vi "NorthWest Window Control_Async.vi"(1 "Desired Window Open %":dbl) -> ()   [LabVIEW 2017]
uses:
  Anemometry/Anemometry Sub Vis/Globals/Dynamic_call_global.ph.vi
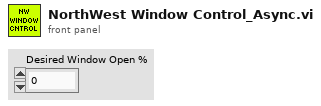
[diagram p1: front panel]
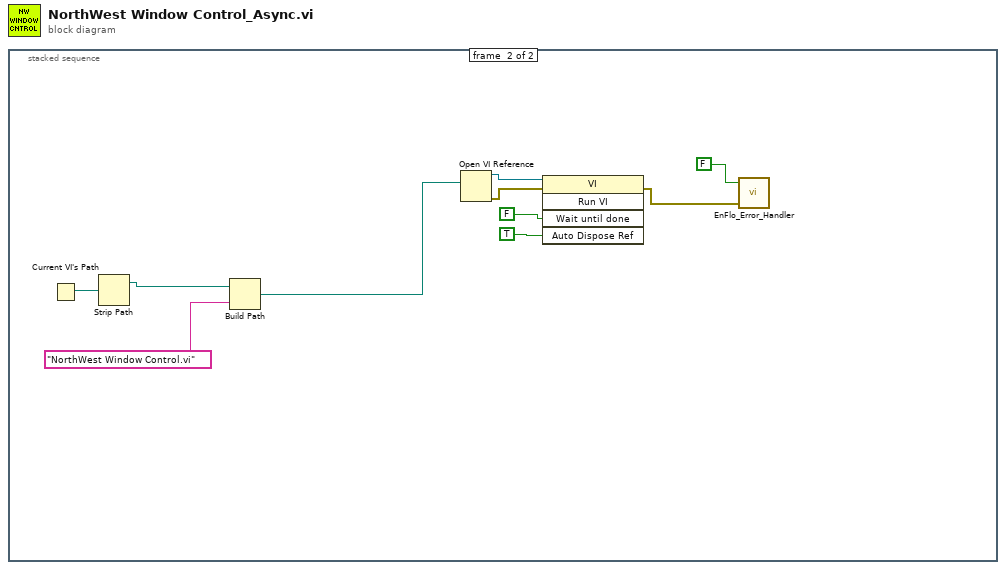
[diagram p0: block diagram]
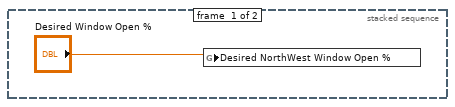
[diagram p2: hidden frame]
diagram:
  n1 = stacked-sequence {
    frame #0 {
      n2 = global write "Dynamic_call_global.ph.vi" "Desired NorthWest Window Open %"("Desired Window Open %") -> ()
    }
    frame #1 {
      n3 = Current VI's Path() -> (path=w7:path)
      n4 = Strip Path(path=w7) -> (stripped path=w6:path)  [unwired: 1 out]
      n5 = Build Path(base path=w6, name or relative path="NorthWest Window Control.vi") -> (appended path=w4:path)
      n6 = Open VI Reference(vi path=w4) -> (vi reference=w9:refnum<vi>, error out=w8:errorcluster)  [unwired: 1 in, 4 out]
      n7 = invoke class="VI" method="Run VI"(reference=w9, error in=w8, "Wait until done"=FALSE, "Auto Dispose Ref"=TRUE) -> (error out=w3:errorcluster)  [unwired: 1 in, 4 out]
      n8 = call "EnFlo_Error_Handler.vi"("error in (no error)"=w3, "Dialog Box (T)"=FALSE) -> ()  [unwired: 1 in, 3 out]
    }
  }
